vi "calculate_phi.vi"(8 "Error In":errorcluster, 10 "xi":dbl, 11 "gamma":dbl) -> (0 "Error Out":errorcluster, 3 "phi":dbl)   [LabVIEW 2019]
doc: "Calculate phi from formula 4 in Wilen(2000). All inputs and outputs are in degrees."
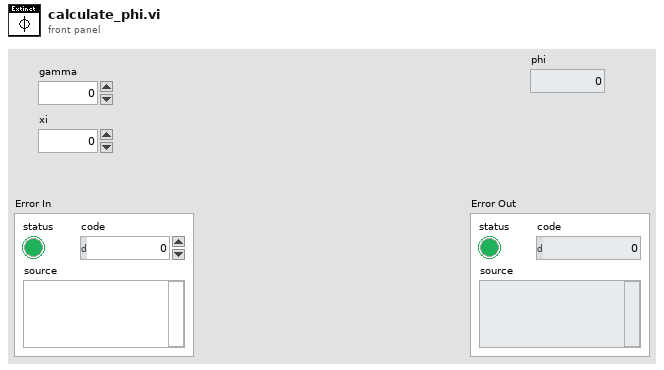
[diagram p1: front panel]
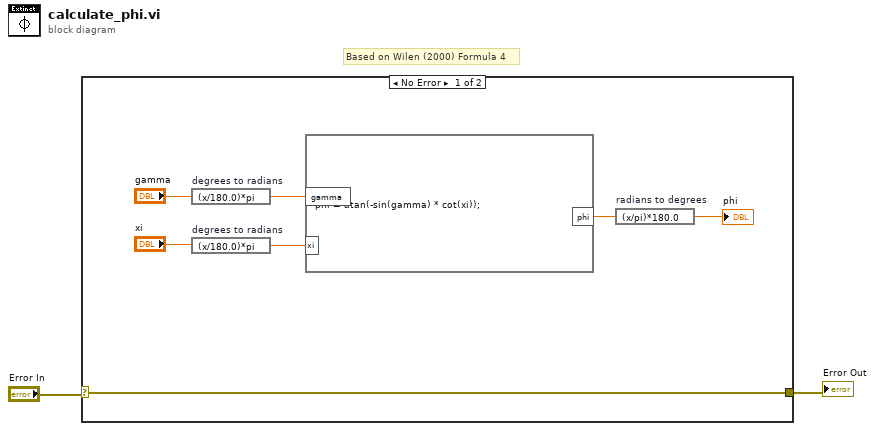
[diagram p0: block diagram]
diagram:
  # "Based on Wilen (2000) Formula 4"
  n1 = case shown="No Error" "Error In" {
    selector: "Error In" -> [w9 w10]
    tunnel: [w9 w10] -> w1
    frame No Error {
      n2 = expression code="(x/180.0)*pi" "degrees to radians"("gamma") -> (w8:dbl)
      n3 = expression code="(x/180.0)*pi" "degrees to radians"("xi") -> (w7:dbl)
      n4 = formula code="phi = atan(-sin(gamma) * cot(xi));"("gamma"=w8, "xi"=w7) -> ("phi"=w6:dbl)
      n5 = expression code="(x/pi)*180.0" "radians to degrees"(w6) -> (→"phi":dbl)
    }
    frame Error {
    }
  }
  "Error Out" <- w1
